vi "to binary.vi"(8 "error in":errorcluster, 11 "byte":u8[](array[numeric]) format="%b") -> (0 "error out":errorcluster, 3 "String":string)   [LabVIEW 2020, in "wamplv.lvlib" / "MessagePack.lvclass"]
uses:
  MessagePack.lvclass
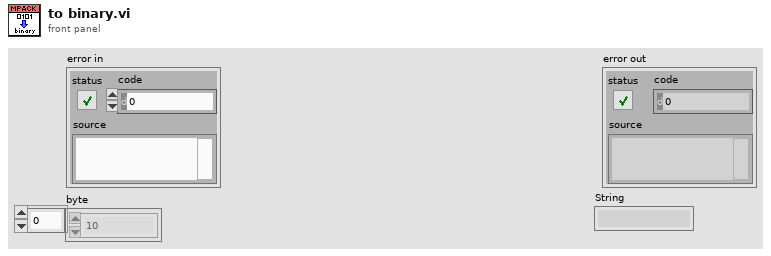
[diagram p1: front panel]
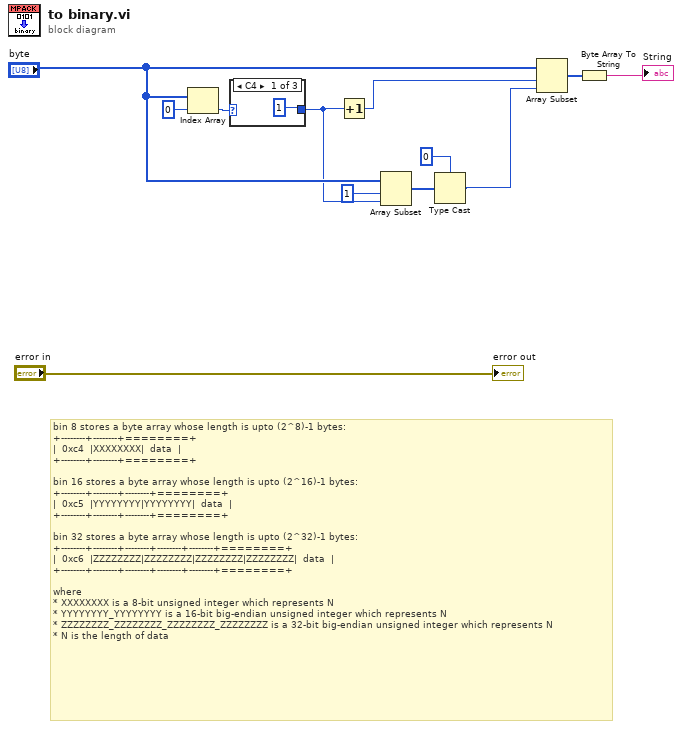
[diagram p0: block diagram]
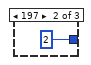
[diagram p2: hidden frame]
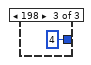
[diagram p3: hidden frame]
diagram:
  # "bin 8 stores a byte array whose length is upto (2^8)-1 bytes:\n+--------+--------+========+\n|  0xc4  |XXXXXXXX|  data  |\n+--------+--------+========+\n\nbin 16 stores a byte array whose length is upto (2^16)-1 bytes:\n+--------+--------+--------+========+\n|  0xc5  |YYYYYYYY|YYYYYYYY|  data  |\n+--------+--------+--------+========+\n\nbin 32 stores a byte array whose length is upto (2^32)-1 bytes:\n+--------+--------+--------+--------+--------+========+\n|  0xc6  |ZZZZZZZZ|ZZZZZZZZ|ZZZZZZZZ|ZZZZZZZZ|  data  |\n+--------+--------+--------+--------+--------+========+\n\nwhere\n* XXXXXXXX is a 8-bit unsigned integer which represents N\n* YYYYYYYY_YYYYYYYY is a 16-bit big-endian unsigned integer which represents N\n* ZZZZZZZZ_ZZZZZZZZ_ZZZZZZZZ_ZZZZZZZZ is a 32-bit big-endian unsigned integer which represents N\n* N is the length of data"
  n1 = Index Array(array="byte", index=0) -> (element=w10:u8)
  n2 = case shown="C4" w10 {
    tunnel: [1 2 4] -> w2
    frame 196 {
    }
    frame 197 {
    }
    frame 198 {
    }
  }
  n3 = Increment(x=w2) -> (x+1=w1:i32)
  n4 = Array Subset(array="byte", index=1, length=w2) -> (w4:u8[])
  n5 = Type Cast(type=u32 0, x=w4) -> (*(type *) &x=w9:u32)
  n6 = Array Subset(array="byte", index=w1, length=w9) -> (w8:u8[])
  n7 = Byte Array To String(unsigned byte array=w8) -> (string=→"String":string)
  "error out" <- "error in"
